vi "linepic.vi"(9 "origin":cluster{"x":dbl, "y":dbl}, 10 "Cluster":cluster{"x":dbl, "y":dbl}, 11 "shift pic":picture) -> (3 "2D Picture 2":picture)   [LabVIEW 2024]
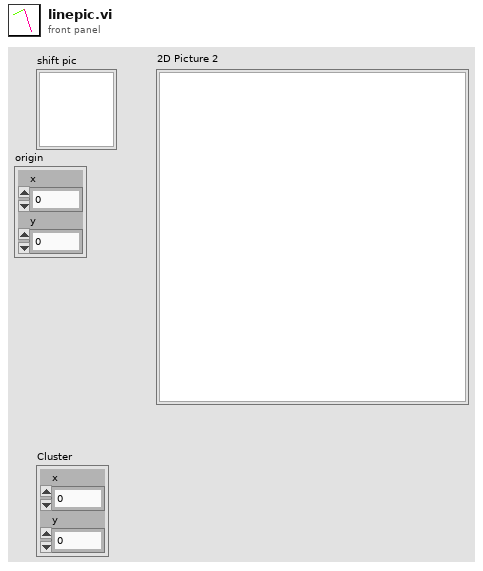
[diagram p1: front panel]
types:
  T1 = cluster{"Width":u16, "Style":enum32{"Solid", "Dash", "Dot", "DashDot", "DashDotDot"}}
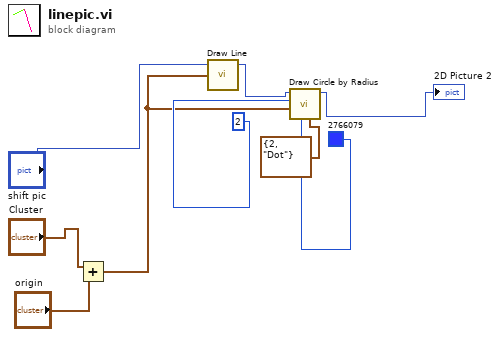
[diagram p0: block diagram]
diagram:
  n1 = Add(x="Cluster", y="origin") -> (x+y=w2:cluster{"x":dbl, "y":dbl})
  n2 = call <vilib>:"Draw Line.vi"("picture"="shift pic", "end point"=w2) -> ("new picture"=w9:picture)  [unwired: 7 in]
  n3 = call <vilib>:"Draw Circle by Radius.vi"("pen"=T1 {"Width"=2, "Style"=enum."Dot"}, "color(black)"=u32 2766079, "pixel center"=w2, "radius"=u16 2 ("Width"), "picture"=w9) -> ("new picture"=→"2D Picture 2":picture)  [unwired: 6 in]
